vi "List NICs.vi"(8 "Error In":errorcluster, 10 "Network Interface Config":string, 11 "ifconfig":string="\neth0      Link encap:Ethernet  HWaddr d0:5f:b8:a3:99:8b\n          inet addr:10.2.229.42  Bcast:10.2.229.255  Mask:255.255.255.0\n          inet6 addr: fe80::d25f:b8ff:fea3:998b/64 Scope:Link\n          UP BROADCAST RUNNING MULTICAST DYNAMIC  MTU:1500  Metric:1\n          RX packets:838912 errors:0 dropped:21264 overruns:0 frame:0\n          TX packets:9842 errors:0 dropped:0 overruns:0 carrier:0\n          collisions:0 txqueuelen:1000\n          RX bytes:107060267 (102.1 MiB)  TX bytes:755097 (737.3 KiB)\n          Interrupt:177\n\nlo        Link encap:Local Loopback\n          inet addr:127.0.0.1  Mask:255.0.0.0\n          inet6 addr: ::1/128 Scope:Host\n          UP LOOPBACK RUNNING  MTU:65536  Metric:1\n          RX packets:378 errors:0 dropped:0 overruns:0 frame:0\n          TX packets:378 errors:0 dropped:0 overruns:0 carrier:0\n          collisions:0 txqueuelen:0\n          RX bytes:30398 (29.6 KiB)  TX bytes:30398 (29.6 KiB)\n\nusb0      Link encap:Ethernet  HWaddr d0:5f:b8:a3:99:80\n          inet addr:192.168.7.2  Bcast:192.168.7.3  Mask:255.255.255.252\n          inet6 addr: fe80::d25f:b8ff:fea3:9980/64 Scope:Link\n          UP BROADCAST RUNNING MULTICAST  MTU:1500  Metric:1\n          RX packets:38659 errors:0 dropped:0 overruns:0 frame:0\n          TX packets:1822 errors:0 dropped:0 overruns:0 carrier:0\n          collisions:0 txqueuelen:1000\n          RX bytes:12819260 (12.2 MiB)  TX bytes:500040 (488.3 KiB)\n") -> (0 "Error Out":errorcluster, 3 "All NICs":string[](array[string]))   [LabVIEW 2019, in "LMH-LINX.lvlib"]
uses:
  <vilib>/MakerHub/LINX/LMH-LINX.lvlib
  <vilib>/regexp/Match Regular Expression.xnode
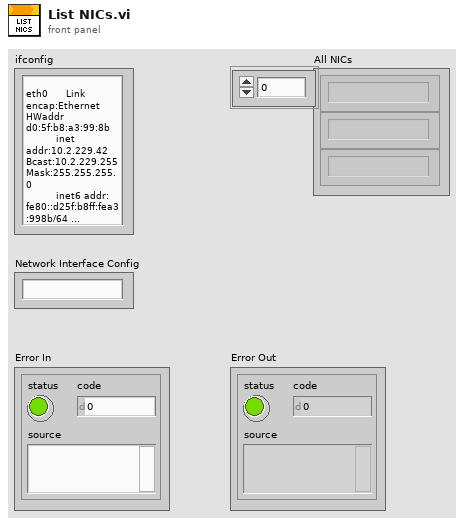
[diagram p1: front panel]
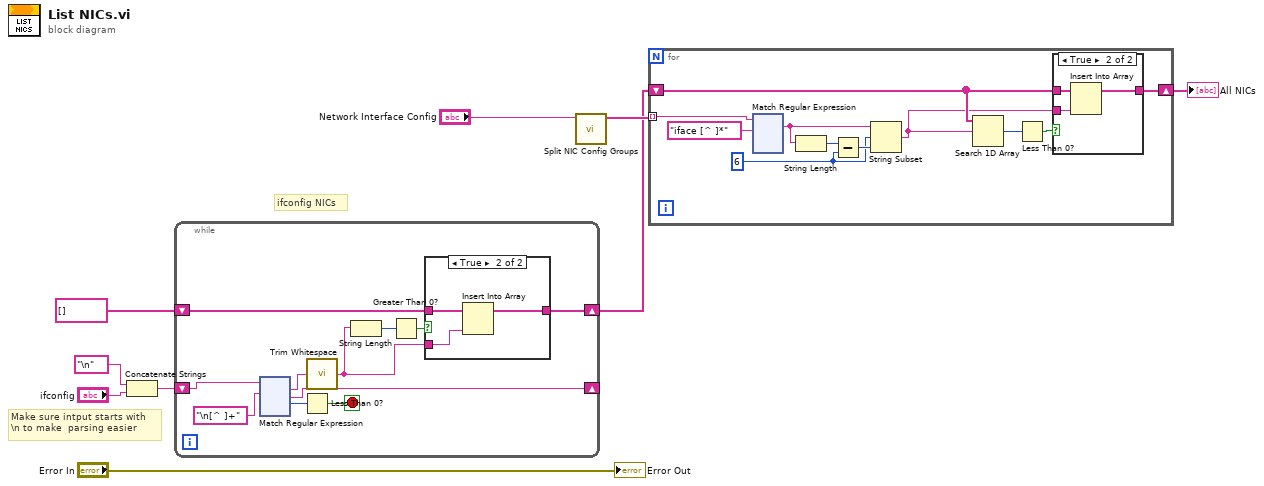
[diagram p0: block diagram]
diagram:
  # "ifconfig NICs"
  # "Make sure intput starts with \n\\n to make  parsing easier"
  n1 = Concatenate Strings("\n", "ifconfig") -> (w6:string)
  n2 = while {
    shift-right: [w15] -> _
    shift-left: w6 -> [w20]
    shift-right: [w10] -> w2
    shift-left: string[] [] -> [w12]
    stop <- w17 stop-if-true
    n3 = xnode "Match Regular Expression"("input string"=w20, "regular expression"="\n[^ ]+") -> ("whole match"=w16:string, "after match"=w15:string, "offset past match"=w18:i32)  [unwired: 4 in, 2 out]
    n4 = Less Than 0?(x=w18) -> (x < 0?=w17:bool)
    n5 = call <vilib>:"Trim Whitespace.vi"("string"=w16) -> ("trimmed string"=w11:string)  [unwired: 1 in]
    n6 = String Length(string=w11) -> (length=w13:i32)
    n7 = Greater Than 0?(x=w13) -> (x > 0?=w14:bool)
    n8 = case shown="True" w14 {
      tunnel: w12 -> [w21 w24]
      tunnel: w11 -> [_ w23]
      tunnel: [w21 w22] -> w10
      frame False {
        # "Empty String\nIgnore"
      }
      frame True {
        n9 = Insert Into Array(array=w24, new element=w23) -> (w22:string[])  [unwired: 1 in]
      }
    }
  }
  n10 = call <vilib>:"Split NIC Config Groups.vi"("Network Interface Config"="Network Interface Config") -> ("NIC Config Groups"=w3:string[])  [unwired: 10 in]
  n11 = for {
    tunnel: w3 -> [w141] mode=indexing
    shift-right: [w136] -> w1
    shift-left: w2 -> [w140]
    w142 = 6 ("y")
    n12 = xnode "Match Regular Expression"("input string"=w141, "regular expression"="iface [^ ]*") -> ("whole match"=w143:string)  [unwired: 4 in, 4 out]
    n13 = String Length(string=w143) -> (length=w145:i32)
    n14 = Subtract(x=w145, y=w142) -> (x-y=w144:i32)
    n15 = String Subset(string=w143, offset (0)=w142, length (rest)=w144) -> (substring=w137:string)
    n16 = Search 1D Array(1D array=w140, element=w137) -> (index of element=w139:i32)  [unwired: 1 in]
    n17 = Less Than 0?(x=w139) -> (x < 0?=w138:bool)
    n18 = case shown="True" w138 {
      tunnel: w140 -> [w147 w150]
      tunnel: w137 -> [_ w149]
      tunnel: [w147 w148] -> w136
      frame False {
      }
      frame True {
        n19 = Insert Into Array(array=w150, new element=w149) -> (w148:string[])  [unwired: 1 in]
      }
    }
  }
  "All NICs" <- w1
  "Error Out" <- "Error In"
